vi "SwerveShortestTurnAlg.vi"(8 "SwerveMotorsFlipped?":bool, 9 "SwerveSpeed":dbl, 10 "AngleSetpoint":dbl, 11 "AngleEncoder":dbl) -> (2 "FlipSwerveMotors":bool, 3 "PIDInput":dbl)   [LabVIEW 2017]
uses:
  SwerveGlobals.vi
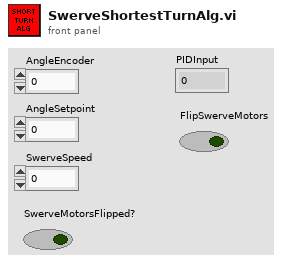
[diagram p1: front panel]
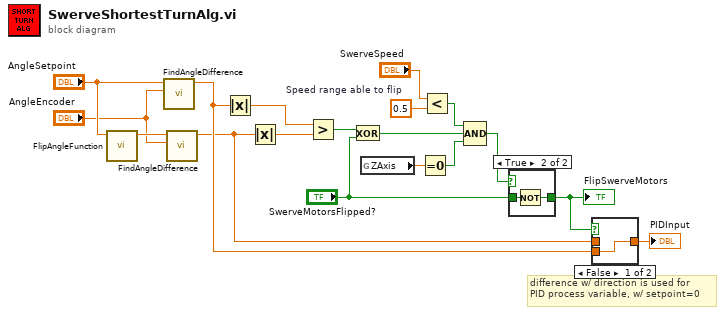
[diagram p0: block diagram]
diagram:
  w18 = 0.5  # Speed range able to flip
  # "difference w/ direction is used for\nPID process variable, w/ setpoint=0"
  n1 = call "FlipAngleFunction.vi"("AngleInput"="AngleSetpoint") -> ("AngleFlipped"=w2:dbl)  [unwired: 10 in]
  n2 = call "FindAngleDifference.vi"("AngleEncoder"="AngleEncoder", "AngleSetpoint"="AngleSetpoint") -> ("Distance/DirectionOfTurn"=w7:dbl)  [unwired: 9 in]
  n3 = call "FindAngleDifference.vi"("AngleEncoder"="AngleEncoder", "AngleSetpoint"=w2) -> ("Distance/DirectionOfTurn"=w3:dbl)  [unwired: 9 in]
  n4 = Absolute Value(x=w7) -> (abs(x)=w6:dbl)
  n5 = Absolute Value(x=w3) -> (abs(x)=w5:dbl)
  n6 = Greater?(x=w6, y=w5) -> (0:w15:bool)
  n7 = Exclusive Or(1:"SwerveMotorsFlipped?", 2:w15) -> (0:w12:bool)
  n8 = global read "SwerveGlobals.vi" "ZAxis"() -> (w17:dbl)
  n9 = Equal To 0?(x=w17) -> (x = 0?=w11:bool)
  n10 = Less?(x="SwerveSpeed", y=w18) -> (x < y?=w13:bool)
  n11 = Compound Arithmetic op=AND(w13, w12, w11) -> (w10:bool)
  n12 = case shown="True" w10 {
    tunnel: "SwerveMotorsFlipped?" -> [w19 w21]
    tunnel: [w19 w20] -> w9
    frame False {
    }
    frame True {
      n13 = Not(x=w21) -> (.not. x?=w20:bool)
    }
  }
  "FlipSwerveMotors" <- w9
  n14 = case shown="False" w9 {
    tunnel: w7 -> [w22 _]
    tunnel: w3 -> [_ w23]
    tunnel: [w22 w23] -> w8
    frame False {
    }
    frame True {
    }
  }
  "PIDInput" <- w8
